vi "New Targets Message.vi"() -> (0 "Vision Message":T1)   [LabVIEW 2016]
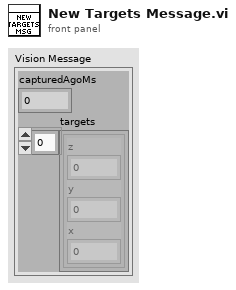
[diagram p1: front panel]
types:
  T1 = cluster{"capturedAgoMs":i32, "targets":cluster{"z":dbl, "y":dbl, "x":dbl}[]}
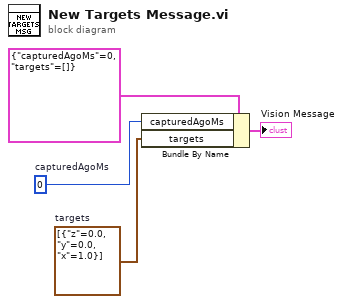
[diagram p0: block diagram]
diagram:
  w2 = cluster{"z":dbl, "y":dbl, "x":dbl}[] [{"z"=0.0, "y"=0.0, "x"=1.0}]  # targets
  w3 = 0  # capturedAgoMs
  n1 = Bundle By Name(cluster=T1 {"capturedAgoMs"=0, "targets"=[]} ("Targets Message"), "capturedAgoMs"=w3, "targets"=w2) -> (→"Vision Message":T1)
